vi "pyexample2.vi"() -> ()   [LabVIEW 2022 SP3]
uses:
  C:/Program Files (x86)/National Instruments/LabVIEW 2022/examples/Connectivity/Python/support/PythonVersionsEnum.ctl
panel:
  out "return value 2":string
  out "Numeric":dbl
  out "return value":bool
  in  "module path":path=path "V:/GitHub/SmartMachine/manager/ex_async_que.py"
  out "error out":errorcluster
  in  "error in (no error)":errorcluster
  in  "python version":T1=enum."3.9"
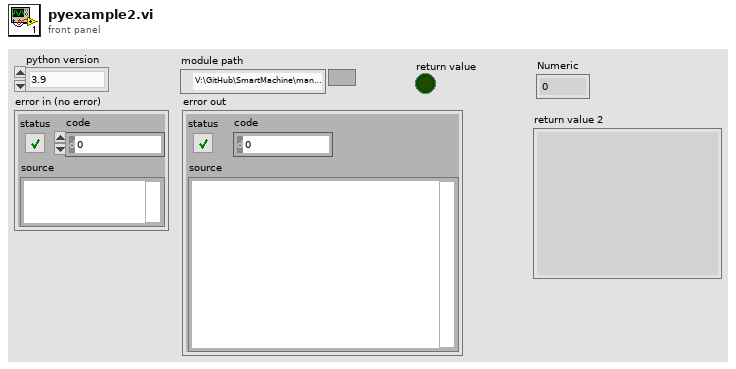
[diagram p1: front panel]
types:
  T1 = typedef "PythonVersionsEnum.ctl" = enum16{"3.6", "3.7", "3.8", "3.9"}
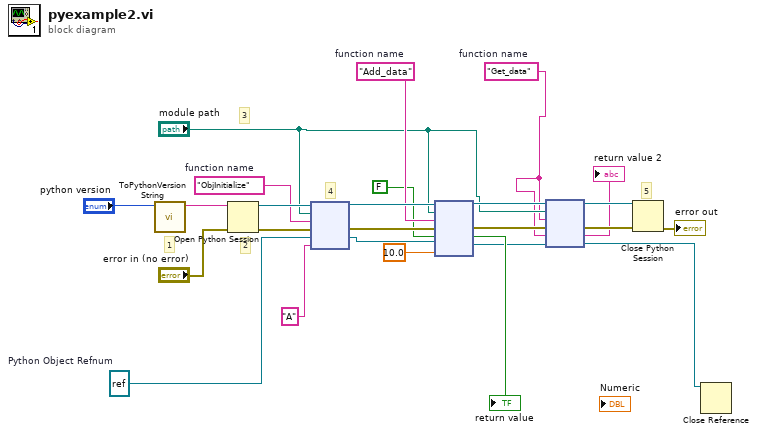
[diagram p0: block diagram]
diagram:
  w2 = "Get_data"  # function name
  w14 = "Add_data"  # function name
  w18 = refnum<k38> refnum  # Python Object Refnum
  w20 = "ObjInitialize"  # function name
  # "5"
  # "4"
  # "2"
  # "3"
  # "1"
  n1 = call "ToPythonVersionString.vi"("python version"="python version") -> ("python version string"=w25:string)  [unwired: 10 in]
  n2 = Open Python Session(python version=w25, 3:"error in (no error)") -> (session out=w22:refnum<k35>, error out=w21:errorcluster)  [unwired: 1 in]
  n3 = node(w22, "module path", w20, w21, w18, "A") -> (w16:refnum<k35>, w17:errorcluster, w15:refnum<k38>)  [unwired: 1 in, 2 out]
  n4 = node(w16, "module path", w14, w17, FALSE, w15, 10.0) -> (w9:refnum<k35>, w6:errorcluster, →"return value":bool, w5:refnum<k38>)  [unwired: 1 in, 2 out]
  n5 = node(w9, "module path", w2, w6, w2, w5) -> (w8:refnum<k35>, w7:errorcluster, →"return value 2":string, w3:refnum<k38>)  [unwired: 2 out]
  n6 = Close Python Session(session in=w8, error in=w7) -> (11:→"error out":errorcluster)
  n7 = Close Reference(reference=w3) -> ()  [unwired: 1 in, 1 out]
